vi "Version.vi"(8 "error in (no error)":errorcluster, 11 "SRV In":refnum<k5>) -> (0 "error out":errorcluster, 1 "Reply":string, 2 "Version":dbl, 3 "SRV Out":refnum<k5>)   [LabVIEW 2009]
doc: "Requests and returns the firmware version.\n\n\nWritten for Benilde St. Margaret's School - Tim Jump\nBy Doug Schmertman - Logic PD\nCopyright 2012"
panel:
  # "This LabVIEW item is deprecated.\n\nIt is believed to be unused and will be removed in a future version of SRV."
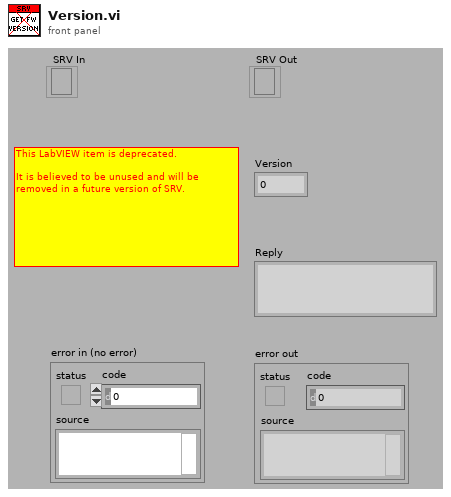
[diagram p1: front panel]
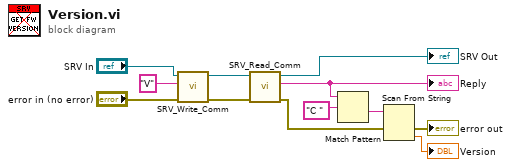
[diagram p0: block diagram]
diagram:
  n1 = call "SRV_Write_Comm.vi"("error in (no error)"="error in (no error)", "Command Sent"="V", "SRV In"="SRV In") -> ("error out"=w4:errorcluster, "SRV Out"=w12:refnum<k5>)  [unwired: 6 in, 1 out]
  n2 = call "SRV_Read_Comm.vi"("error in (no error)"=w4, "SRV In"=w12) -> ("error out"=w3:errorcluster, "Data out"=w5:string, "SRV Out"=→"SRV Out":refnum<k5>)  [unwired: 7 in]
  "Reply" <- w5
  n3 = Match Pattern(string=w5, regular expression="C " ("Command Sent")) -> (after substring=w7:string)  [unwired: 1 in, 3 out]
  n4 = Scan From String(input string=w7, error in=w3) -> (error out=→"error out":errorcluster, output 1=→"Version":dbl)  [unwired: 3 in, 2 out]
